vi "系统变量.vi"() -> ()   [LabVIEW 2016, in "斯坦道CODMn.lvlib"]
panel:
  in  "运行间隔":i16=4 min=1 max=24
  in  "CODmn":dbl
  in  "总氮":dbl
  in  "总磷":dbl
  in  "氨氮":dbl
  in  "pH":dbl
  in  "水温":dbl
  in  "自动切换量程":bool=TRUE
  in  "运行模式":enum16{"维护模式", "常规模式", "应急模式", "质控模式"}(ring)
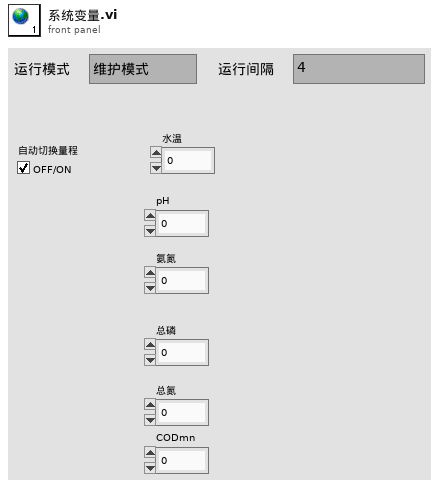
[diagram p1: front panel]
diagram:
